vi "Proiecr_MDA.vi"() -> ()   [LabVIEW 2019]
uses:
  <vilib>/Analysis/Matrix/Datatypes/RealMatrix.ctl
  <vilib>/robotics/Kinematics/DH Kinematic Parameters.ctl
  <vilib>/robotics/Kinematics/Link/Joint Type.ctl
  <vilib>/robotics/Kinematics/NI_Kinematics.lvlib
  <vilib>/robotics/Kinematics/Link/NI_Robotics_Link.lvclass
  <vilib>/Analysis/Matrix/NI_Matrix.lvlib
panel:
  out "3D Picture":refnum<vi>(3d-picture)
  in  "j6":dbl(slide) scale=0.0..6.2831
  in  "j5":dbl(slide) scale=-1.5707..1.5707
  in  "j4":dbl(slide) scale=0.0..6.2831
  in  "j3":dbl(slide) scale=-2.5..2.5
  in  "j2":dbl(slide) scale=-2.17..2.17
  in  "j1":dbl(slide) scale=0.0..6.2831
  out "array to string":string
  in  "index":dbl
  out "Array":cluster{string, "number of columns":i32}[](array[cluster])
  in  "stop":bool
  out "Translation Matrix":T1
  out "Rotation Matrix Fake":T1
  out "Orientation XYZ Fake":dbl[](array[numeric])
  in  "Debug":bool
  in  "?":enum32{"Configuration", "Manipulate", "Points"}(tab)
  in  "j6 L":dbl
  in  "j4 L":dbl
  in  "j5 L":dbl=-1.5707
  in  "j1 L":dbl
  in  "j2 L":dbl=-2.17
  in  "j3 L":dbl=-2.5
  in  "j6 U":dbl=6.2831
  in  "j4 U":dbl=6.2831
  in  "j5 U":dbl=1.5707
  in  "j1 U":dbl=6.2831
  in  "j2 U":dbl=2.17
  in  "j3 U":dbl=2.5
  in  "l1":dbl=1.3
  in  "l2":dbl=2.5
  in  "l3":dbl=1.25
  in  "l4":dbl=1.25
  in  "l5":dbl=1.0
  in  "base":dbl=0.9
  in  "Generate file":bool
  in  "Pause time (sec)":i64=1
  in  "End Spline":bool
  out "Select Trajectory":bool
  out "Loop activ":bool
  in  "Loop":bool
  out "Gripper Closed":bool
  in  "Activate Gripper":bool
  out "Active":bool
  out "End Point":bool
  out "Intermidiate Point":bool
  in  "Spline":bool
  in  "Circle":bool
  in  "Line":bool
  in  "Add Point":bool
  out "RX":dbl
  out "RY":dbl
  out "RZ":dbl
  out "X":dbl
  out "Y":dbl
  out "Z":dbl
  in  "Pause":bool
  out "Real Matrix":T1
  # "Dimensions of the manipulator"
  # "Arm"
  # "Wrist"
  # "Base"
  # "Limits of the joints"
  # "Joint 1"
  # "Joint 2"
  # "Joint 3"
  # "Upper\nLimit"
  # "Lower\nLimit"
  # "Joint 4"
  # "Joint 5"
  # "Joint 6"
  # "Upper\nLimit"
  # "Lower\nLimit"
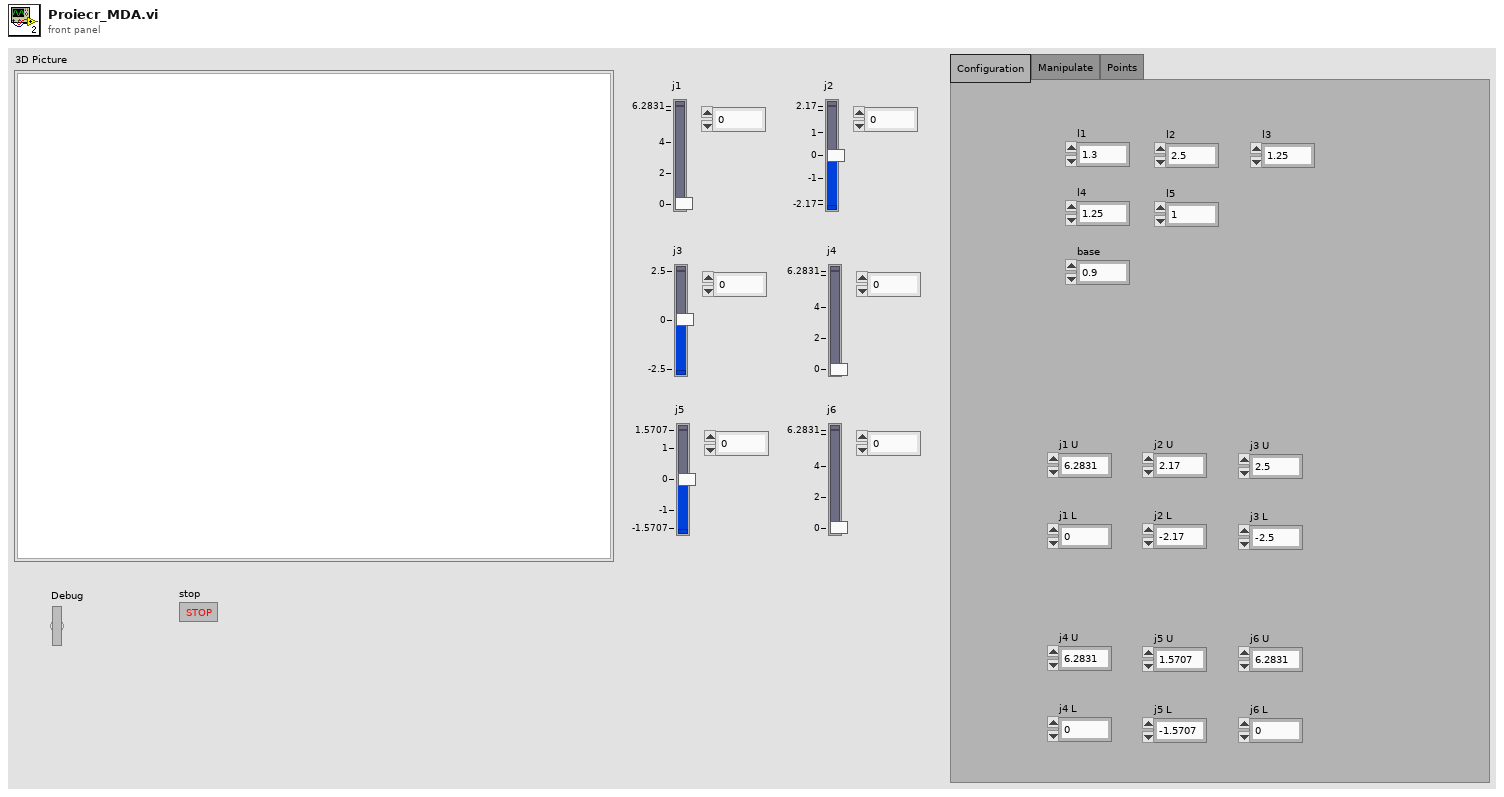
[diagram p1: front panel]
types:
  T1 = typedef "NI_Matrix.lvlib/RealMatrix.ctl" = dbl[][]
  T2 = enum16{"open", "replace", "create", "open or create", "replace or create", "replace or create with confirmation"}
  T3 = enum8{"Enabled", "Disabled", "Disabled and Grayed Out"}
  T4 = typedef "DH Kinematic Parameters.ctl" = cluster{"twist angle":dbl, "length":dbl, "rotation angle":dbl, "offset distance":dbl, "joint type":T5, "joint coordinate offset":dbl}
  T5 = typedef "NI_Robotics_Link.lvclass/Joint Type.ctl" = enum16{"Revolute", "Prismatic"}
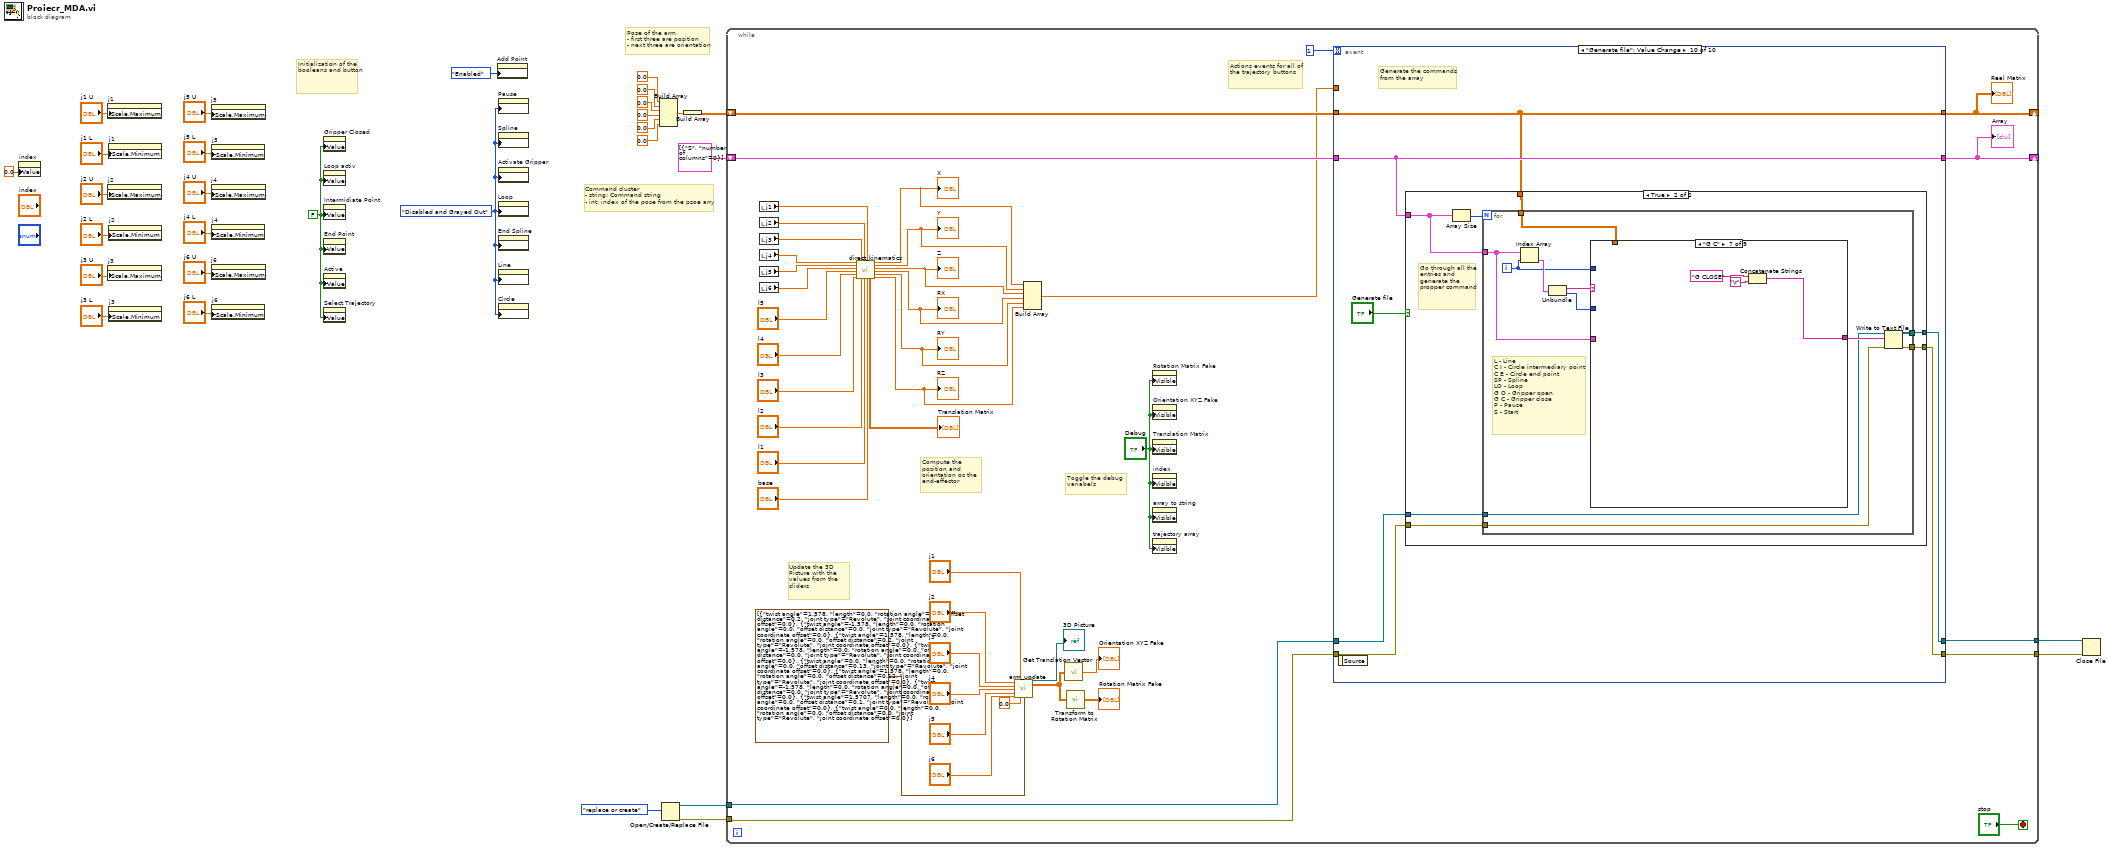
[diagram p0: block diagram]
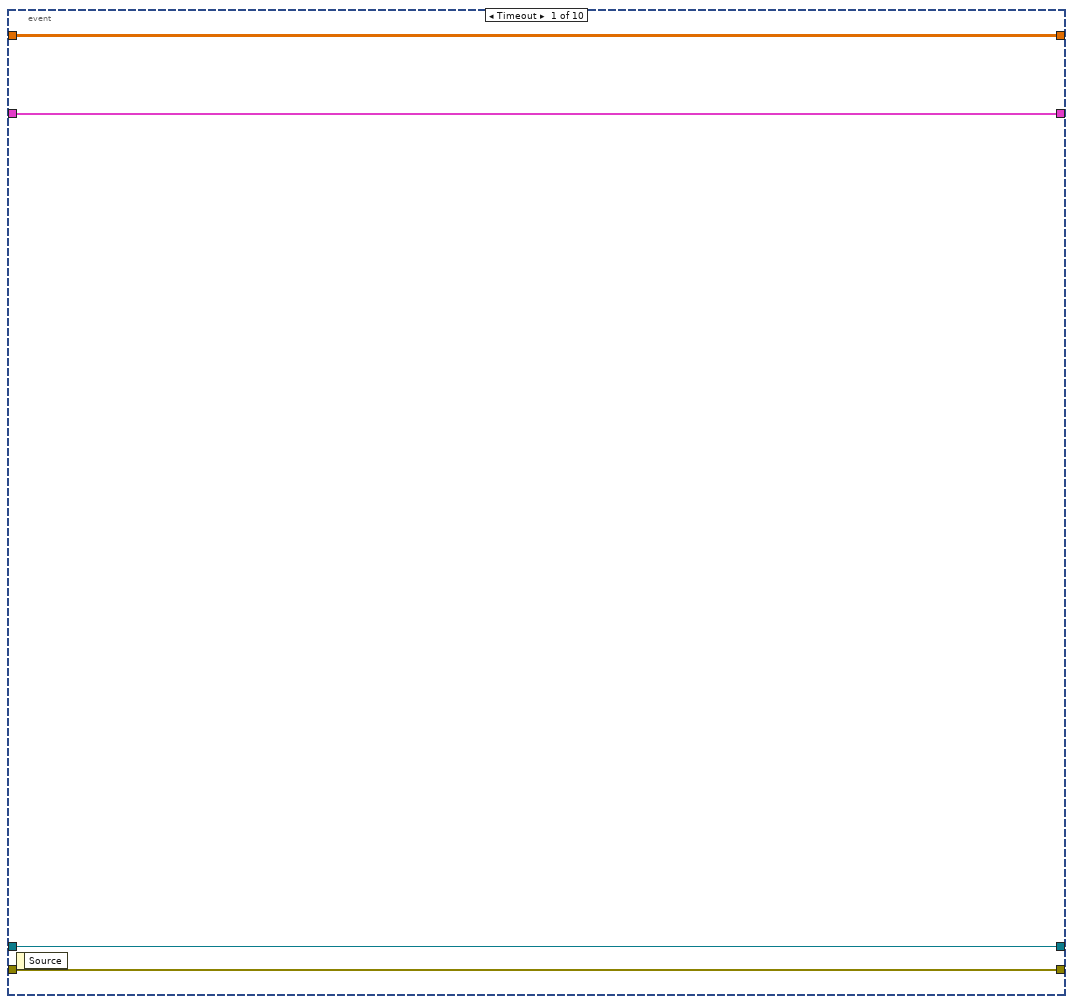
[diagram p2: hidden frame]
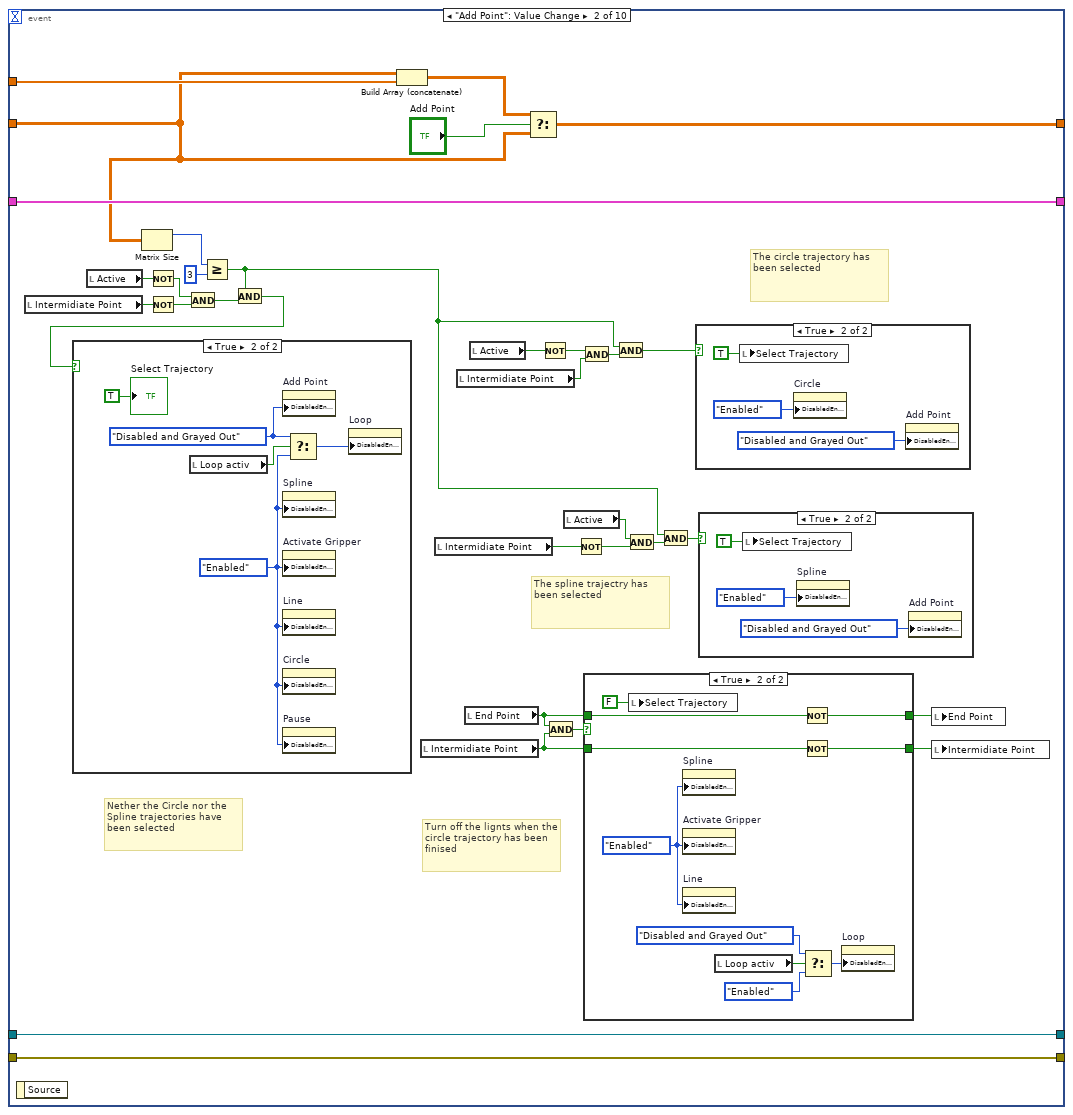
[diagram p3: hidden frame]
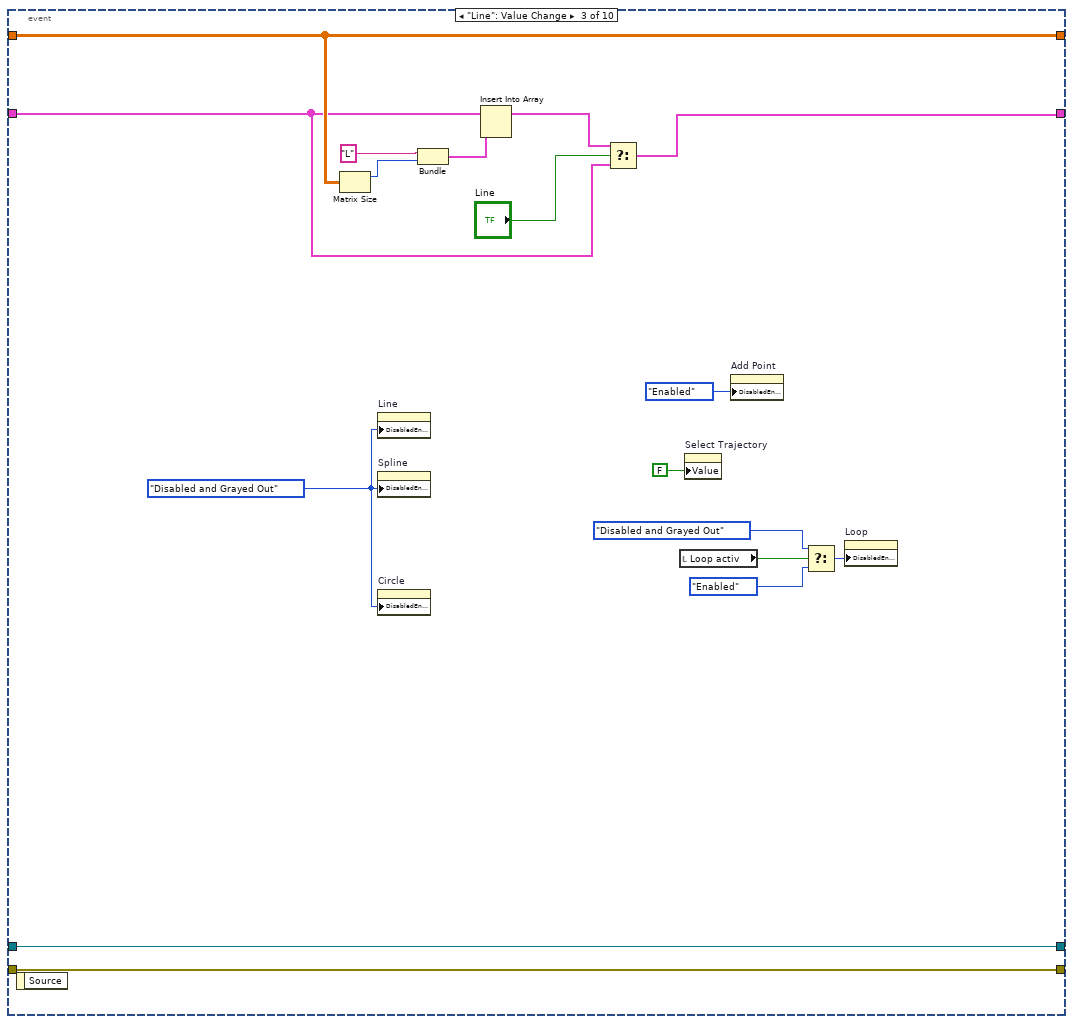
[diagram p8: hidden frame]
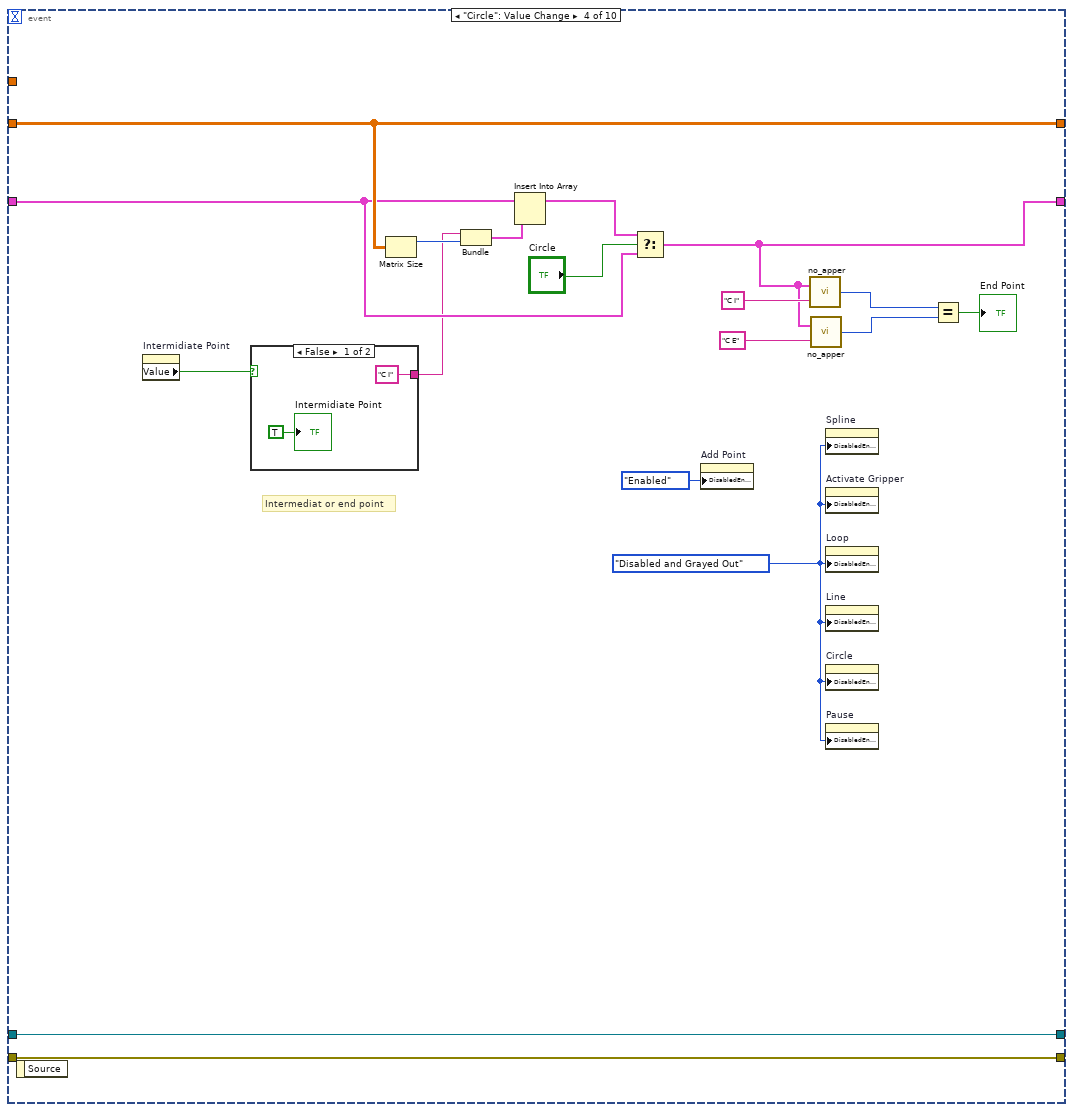
[diagram p9: hidden frame]
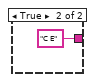
[diagram p10: hidden frame]
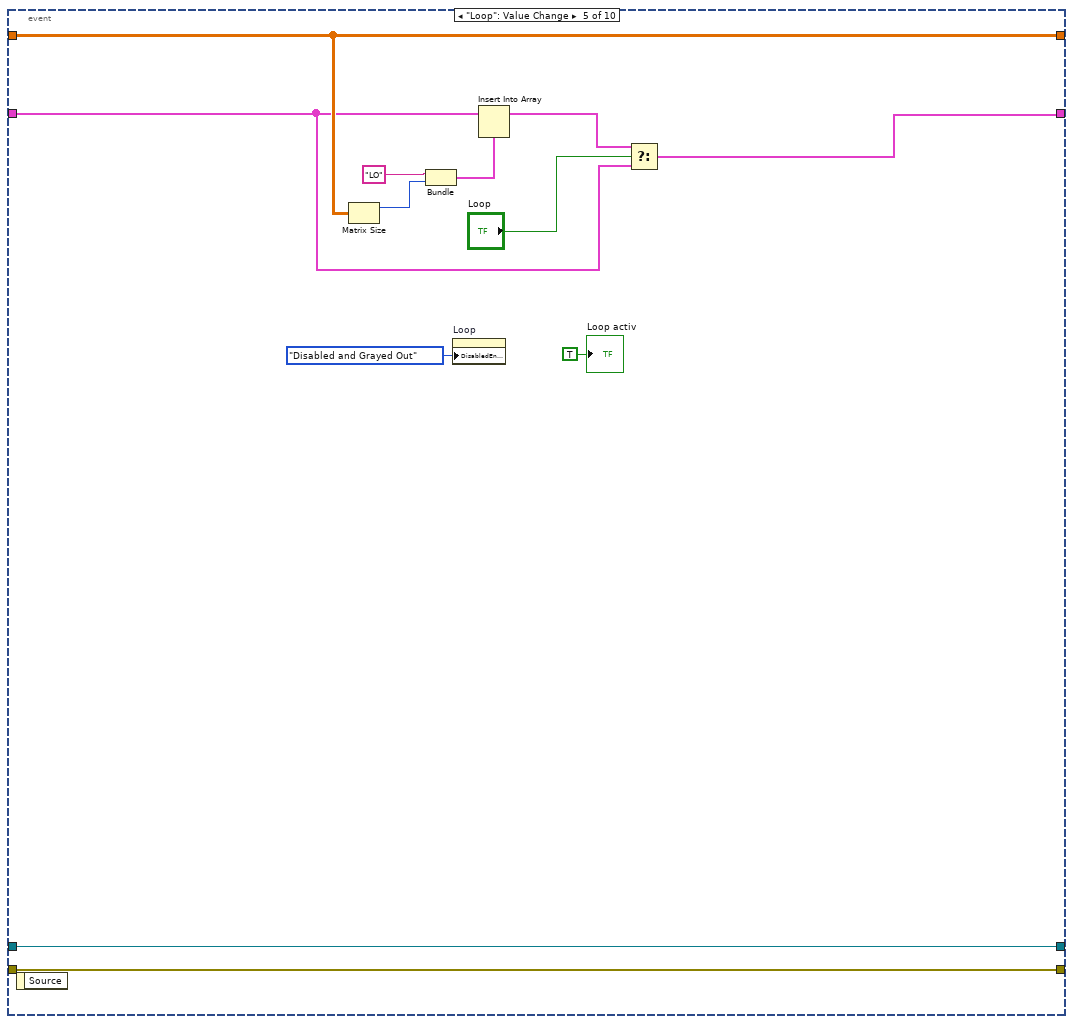
[diagram p11: hidden frame]
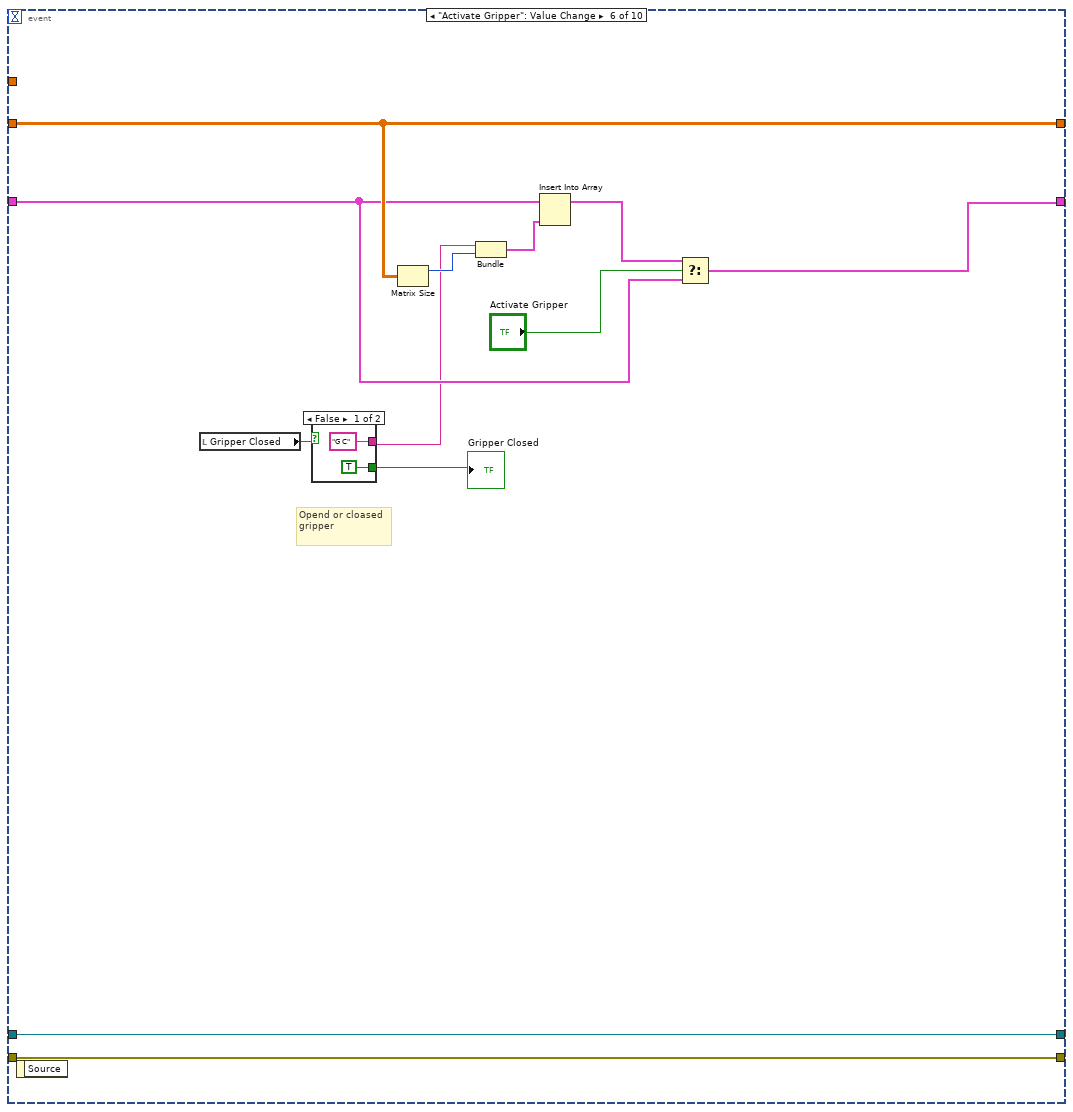
[diagram p12: hidden frame]
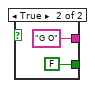
[diagram p13: hidden frame]
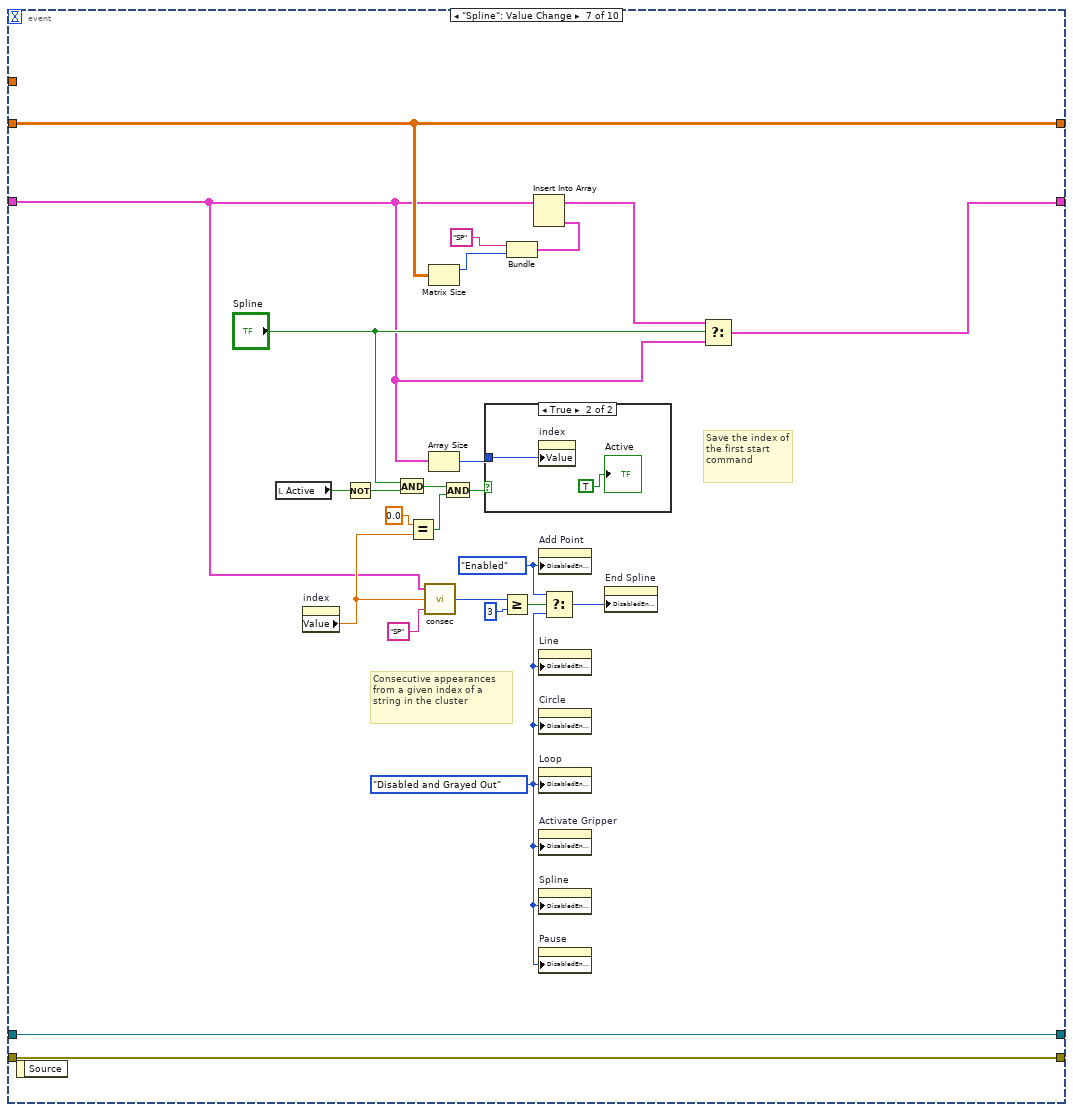
[diagram p14: hidden frame]
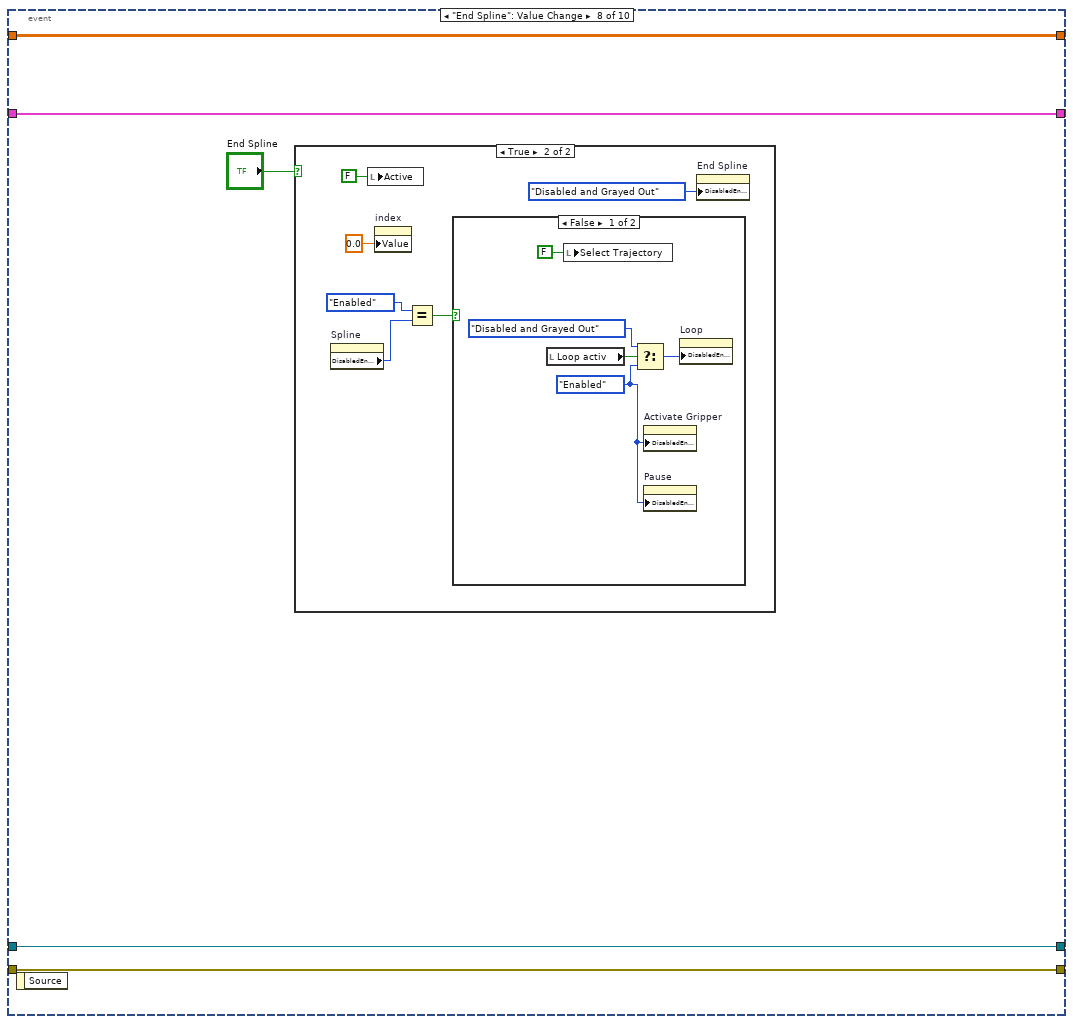
[diagram p16: hidden frame]
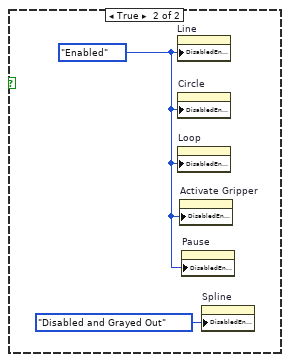
[diagram p18: hidden frame]
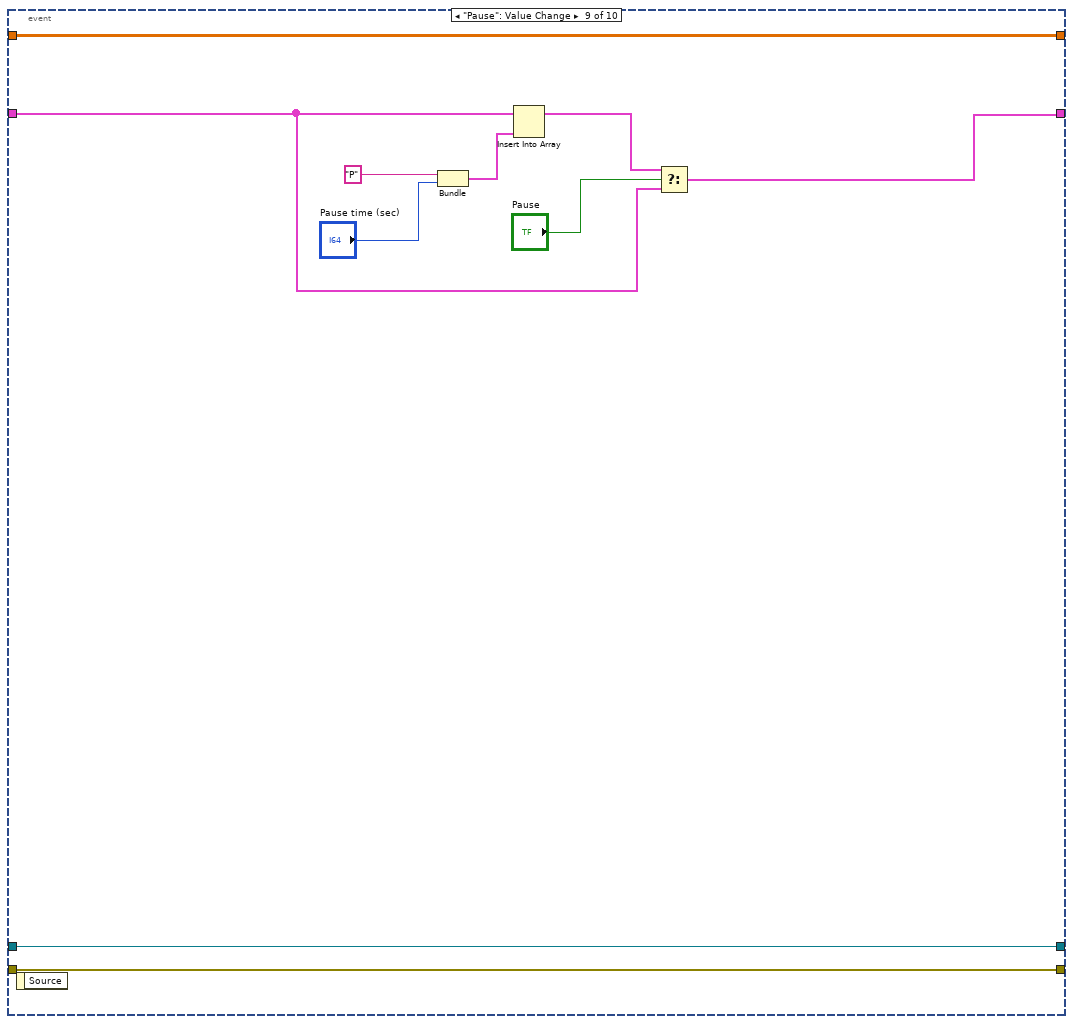
[diagram p19: hidden frame]
diagram:
  w2 = FALSE
  w8 = T3."Disabled and Grayed Out" ("Disabled")
  # "Command cluster \n- string: Command string \n- int: index of the pose from the psoe arry"
  # "Pose of the arm\n- first three are position \n- next three are orientation"
  # "Initialization of the booleans and button"
  n1 = property on="index" class="DigNum (strict)"("Value"=0.0 ("index")) -> ()  [unwired: 2 in, 2 out]
  n2 = property on="j1" class="Slide (strict)"("Scale.Maximum"="j1 U") -> ()  [unwired: 2 in, 2 out]
  n3 = property on="j2" class="Slide (strict)"("Scale.Maximum"="j2 U") -> ()  [unwired: 2 in, 2 out]
  n4 = property on="j3" class="Slide (strict)"("Scale.Maximum"="j3 U") -> ()  [unwired: 2 in, 2 out]
  n5 = property on="j1" class="Slide (strict)"("Scale.Minimum"="j1 L") -> ()  [unwired: 2 in, 2 out]
  n6 = property on="j2" class="Slide (strict)"("Scale.Minimum"="j2 L") -> ()  [unwired: 2 in, 2 out]
  n7 = property on="j3" class="Slide (strict)"("Scale.Minimum"="j3 L") -> ()  [unwired: 2 in, 2 out]
  n8 = property on="j5" class="Slide (strict)"("Scale.Maximum"="j5 U") -> ()  [unwired: 2 in, 2 out]
  n9 = property on="j4" class="Slide (strict)"("Scale.Maximum"="j4 U") -> ()  [unwired: 2 in, 2 out]
  n10 = property on="j6" class="Slide (strict)"("Scale.Maximum"="j6 U") -> ()  [unwired: 2 in, 2 out]
  n11 = property on="j5" class="Slide (strict)"("Scale.Minimum"="j5 L") -> ()  [unwired: 2 in, 2 out]
  n12 = property on="j4" class="Slide (strict)"("Scale.Minimum"="j4 L") -> ()  [unwired: 2 in, 2 out]
  n13 = property on="j6" class="Slide (strict)"("Scale.Minimum"="j6 L") -> ()  [unwired: 2 in, 2 out]
  n14 = property on="Gripper Closed" class="Bool (strict)"("Value"=w2) -> ()  [unwired: 2 in, 2 out]
  n15 = property on="Loop activ" class="Bool (strict)"("Value"=w2) -> ()  [unwired: 2 in, 2 out]
  n16 = property on="Intermidiate Point" class="Bool (strict)"("Value"=w2) -> ()  [unwired: 2 in, 2 out]
  n17 = property on="End Point" class="Bool (strict)"("Value"=w2) -> ()  [unwired: 2 in, 2 out]
  n18 = property on="Active" class="Bool (strict)"("Value"=w2) -> ()  [unwired: 2 in, 2 out]
  n19 = property on="Select Trajectory" class="Bool (strict)"("Value"=w2) -> ()  [unwired: 2 in, 2 out]
  n20 = property on="Add Point" class="Bool (strict)"("DisabledEnum"=T3."Enabled" ("Disabled")) -> ()  [unwired: 2 in, 2 out]
  n21 = property on="Pause" class="Bool (strict)"("DisabledEnum"=w8) -> ()  [unwired: 2 in, 2 out]
  n22 = property on="Spline" class="Bool (strict)"("DisabledEnum"=w8) -> ()  [unwired: 2 in, 2 out]
  n23 = property on="Activate Gripper" class="Bool"("DisabledEnum"=w8) -> ()  [unwired: 2 in, 2 out]
  n24 = property on="Loop" class="Bool (strict)"("DisabledEnum"=w8) -> ()  [unwired: 2 in, 2 out]
  n25 = property on="End Spline" class="Bool (strict)"("DisabledEnum"=w8) -> ()  [unwired: 2 in, 2 out]
  n26 = property on="Line" class="Bool (strict)"("DisabledEnum"=w8) -> ()  [unwired: 2 in, 2 out]
  n27 = property on="Circle" class="Bool (strict)"("DisabledEnum"=w8) -> ()  [unwired: 2 in, 2 out]
  n28 = Build Array(0.0 ("element"), 0.0 ("element"), 0.0 ("element"), 0.0 ("element"), 0.0 ("element"), 0.0 ("element")) -> (w13:dbl[])
  n29 = Open/Create/Replace File(operation (0:open)=T2."replace or create") -> (refnum out=w4:refnum<file>, error out=w5:errorcluster)  [unwired: 5 in, 1 out]
  n30 = Build Array(w13) -> (w12:T1)
  n31 = while {
    shift-right: [w62] -> _
    shift-left: w12 -> [w69]
    shift-right: [w67] -> _
    shift-left: cluster{string, "number of columns":i32}[] [{"S", "number of columns"=0}] -> [w68]
    tunnel: [w66] -> w7
    tunnel: [w65] -> w6
    tunnel: w5 -> [w64]
    tunnel: w4 -> [w63]
    stop <- "stop" stop-if-true
    # "Actions events for all of the trajectory buttons"
    # "Toggle the debug variabels"
    # "Update the 3D Picture with the values from the sliders"
    # "Compute the position and orientation oc the end-effector"
    n32 = local read "j1"() -> (w52:dbl)
    n33 = local read "j2"() -> (w51:dbl)
    n34 = local read "j3"() -> (w50:dbl)
    n35 = local read "j4"() -> (w49:dbl)
    n36 = local read "j5"() -> (w48:dbl)
    n37 = local read "j6"() -> (w47:dbl)
    n38 = call "direct_kinematics.vi"("j4"=w49, "j5"=w48, "j6"=w47, "l5"="l5", "l4"="l4", "l3"="l3", "j3"=w50, "l2"="l2", "j2"=w51, "l1"="l1", "j1"=w52, "base"="base") -> ("Translation Matrix"=→"Translation Matrix":T1, "X"=w39:dbl, "Y"=w38:dbl, "Z"=w37:dbl, "RX"=w36:dbl, "RY"=w35:dbl, "RZ"=w34:dbl)  [unwired: 1 in]
    "RX" <- w36
    "RY" <- w35
    "RZ" <- w34
    "X" <- w39
    "Y" <- w38
    "Z" <- w37
    n39 = call "arm_update.vi"("j2"="j2", "j1"="j1", "j3"="j3", "j4"="j4", "j5"="j5", "j6"="j6", "element"=0.0, "kinematic parameters"=T4[] [{"twist angle"=1.578, "length"=0.0, "rotation angle"=0.0, "offset distance"=0.2, "joint type"=enum."Revolute", "joint coordinate offset"=0.0}, {"twist angle"=-1.578, "length"=0.0, "rotation angle"=0.0, "offset distance"=0.0, "joint type"=enum."Revolute", "joint coordinate offset"=0.0}, {"twist angle"=1.578, "length"=0.0, "rotation angle"=0.0, "offset distance"=0.2, "joint type"=enum."Revolute", "joint coordinate offset"=0.0}, {"twist angle"=-1.578, "length"=0.0, "rotation angle"=0.0, "offset distance"=0.0, "joint type"=enum."Revolute", "joint coordinate offset"=0.0}, {"twist angle"=0.0, "length"=0.0, "rotation angle"=0.0, "offset distance"=0.13, "joint type"=enum."Revolute", "joint coordinate offset"=0.0}, {"twist angle"=1.578, "length"=0.0, "rotation angle"=0.0, "offset distance"=0.12, "joint type"=enum."Revolute", "joint coordinate offset"=0.0}, {"twist angle"=-1.578, "length"=0.0, "rotation angle"=0.0, "offset distance"=0.0, "joint type"=enum."Revolute", "joint coordinate offset"=0.0}, {"twist angle"=1.5707, "length"=0.0, "rotation angle"=0.0, "offset distance"=0.1, "joint type"=enum."Revolute", "joint coordinate offset"=0.0}, {"twist angle"=0.0, "length"=0.0, "rotation angle"=0.0, "offset distance"=0.0, "joint type"=enum."Revolute", "joint coordinate offset"=0.0}]) -> ("SceneObject out"=→"3D Picture":refnum<vi>, "end effector transform"=w53:T1)  [unwired: 6 in]
    n40 = Build Array(w39, w38, w37, w36, w35, w34) -> (w33:dbl[])
    n41 = call <vilib>:"Get Translation Vector.vi"("transform"=w53) -> ("translation vector"=→"Orientation XYZ Fake":dbl[])
    n42 = call <vilib>:"Transform to Rotation Matrix.vi"("transform"=w53) -> ("rotation matrix"=→"Rotation Matrix Fake":T1)
    n43 = property on="Rotation Matrix Fake" class="Arr (strict)"("Visible"="Debug") -> ()  [unwired: 2 in, 2 out]
    n44 = property on="Orientation XYZ Fake" class="Arr (strict)"("Visible"="Debug") -> ()  [unwired: 2 in, 2 out]
    n45 = property on="Translation Matrix" class="Arr (strict)"("Visible"="Debug") -> ()  [unwired: 2 in, 2 out]
    n46 = property on="index" class="DigNum (strict)"("Visible"="Debug") -> ()  [unwired: 2 in, 2 out]
    n47 = property on="array to string" class="Str"("Visible"="Debug") -> ()  [unwired: 2 in, 2 out]
    n48 = property on="trajectory array" class="Arr (strict)"("Visible"="Debug") -> ()  [unwired: 2 in, 2 out]
    n49 = event shown="[9] \"Generate file\": Value Change" {
      selector: _ -> [_ _ _ _ _ _ _ _ _ _]
      dyn-events: _ -> [_ _ _ _ _ _ _ _ _ _]
      timeout: 1 -> [_ _ _ _ _ _ _ _ _ _]
      tunnel: w33 -> [_ w109 _ _ _ _ _ _ _ _]
      tunnel: [w77 w106 w148 w164 w177 w190 w220 w230 w249 w259] -> w62
      tunnel: w69 -> [w77 w78 w148 w164 w177 w190 w220 w230 w249 w259]
      tunnel: w68 -> [w76 w103 w141 w162 w176 w189 w200 w229 w251 w260]
      tunnel: [w76 w103 w142 w150 w174 w191 w221 w229 w250 w260] -> w67
      tunnel: [w74 w79 w133 w157 w171 w183 w201 w226 w244 w258] -> w66
      tunnel: [w75 w80 w134 w158 w172 w184 w202 w227 w245 w257] -> w65
      tunnel: w64 -> [w74 w79 w133 w157 w171 w183 w201 w226 w244 w256]
      tunnel: w63 -> [w75 w80 w134 w158 w172 w184 w202 w227 w245 w255]
      event Timeout {
        n50 = event-data() -> ()  [unwired: 1 in, 1 out]
      }
      event "Add Point": Value Change {
        # "Turn off the lignts when the circle trajectory has been finised"
        # "The spline trajectry has been selected"
        # "The circle trajectory has been selected"
        # "Nether the Circle nor the Spline trajectories have been selected"
        n51 = event-data() -> ()  [unwired: 1 in, 1 out]
        n52 = local read "Intermidiate Point"() -> (w97:bool)
        n53 = local read "Active"() -> (w95:bool)
        n54 = Matrix Size(0:w78) -> (1:w105:i32)  [unwired: 1 out]
        n55 = Not(x=w95) -> (.not. x?=w94:bool)
        n56 = Not(x=w97) -> (.not. x?=w96:bool)
        n57 = And(x=w94, y=w96) -> (x .and. y?=w98:bool)
        n58 = Greater Or Equal?(x=w105, y=3) -> (x >= y?=w83:bool)
        n59 = And(x=w83, y=w98) -> (x .and. y?=w99:bool)
        n60 = case shown="True" w99 {
          frame False {
          }
          frame True {
            w118 = T3."Disabled and Grayed Out" ("Disabled")
            w116 = T3."Enabled" ("Disabled")
            n61 = local read "Loop activ"() -> (w119:bool)
            n62 = property on="Add Point" class="Bool (strict)"("DisabledEnum"=w118) -> ()  [unwired: 2 in, 2 out]
            n63 = property on="Spline" class="Bool (strict)"("DisabledEnum"=w116) -> ()  [unwired: 2 in, 2 out]
            n64 = property on="Activate Gripper" class="Bool"("DisabledEnum"=w116) -> ()  [unwired: 2 in, 2 out]
            n65 = property on="Line" class="Bool (strict)"("DisabledEnum"=w116) -> ()  [unwired: 2 in, 2 out]
            n66 = property on="Circle" class="Bool (strict)"("DisabledEnum"=w116) -> ()  [unwired: 2 in, 2 out]
            n67 = property on="Pause" class="Bool (strict)"("DisabledEnum"=w116) -> ()  [unwired: 2 in, 2 out]
            n68 = Select(t=w118, s=w119, f=w116) -> (s? t:f=w117:T3)
            n69 = property on="Loop" class="Bool (strict)"("DisabledEnum"=w117) -> ()  [unwired: 2 in, 2 out]
            "Select Trajectory" <- TRUE ("Select Trajectory")
          }
        }
        n70 = Build Array (concatenate)(w78, w109) -> (w107:T1)
        n71 = local read "Intermidiate Point"() -> (w82:bool)
        n72 = local read "Intermidiate Point"() -> (w88:bool)
        n73 = local read "Intermidiate Point"() -> (w91:bool)
        n74 = local read "End Point"() -> (w81:bool)
        n75 = local read "Active"() -> (w93:bool)
        n76 = Select(t=w107, s="Add Point", f=w78) -> (s? t:f=w106:T1)
        n77 = Not(x=w93) -> (.not. x?=w92:bool)
        n78 = And(x=w81, y=w82) -> (x .and. y?=w102:bool)
        n79 = local read "Active"() -> (w87:bool)
        n80 = Not(x=w88) -> (.not. x?=w86:bool)
        n81 = And(x=w92, y=w91) -> (x .and. y?=w90:bool)
        n82 = case shown="True" w102 {
          tunnel: w82 -> [w122 w132]
          tunnel: w81 -> [w121 w131]
          tunnel: [w121 w130] -> w101
          tunnel: [w122 w129] -> w100
          frame False {
          }
          frame True {
            w127 = T3."Enabled" ("Disabled")
            n83 = local write "Select Trajectory"(FALSE) -> ()
            n84 = property on="Spline" class="Bool (strict)"("DisabledEnum"=w127) -> ()  [unwired: 2 in, 2 out]
            n85 = property on="Activate Gripper" class="Bool"("DisabledEnum"=w127) -> ()  [unwired: 2 in, 2 out]
            n86 = property on="Line" class="Bool (strict)"("DisabledEnum"=w127) -> ()  [unwired: 2 in, 2 out]
            n87 = local read "Loop activ"() -> (w126:bool)
            n88 = Not(x=w131) -> (.not. x?=w130:bool)
            n89 = Not(x=w132) -> (.not. x?=w129:bool)
            n90 = Select(t=T3."Disabled and Grayed Out" ("Disabled"), s=w126, f=T3."Enabled" ("Disabled")) -> (s? t:f=w123:T3)
            n91 = property on="Loop" class="Bool (strict)"("DisabledEnum"=w123) -> ()  [unwired: 2 in, 2 out]
          }
        }
        n92 = And(x=w83, y=w90) -> (x .and. y?=w89:bool)
        n93 = And(x=w87, y=w86) -> (x .and. y?=w84:bool)
        n94 = And(x=w83, y=w84) -> (x .and. y?=w85:bool)
        n95 = case shown="True" w89 {
          frame False {
          }
          frame True {
            n96 = local write "Select Trajectory"(TRUE ("Select Trajectory")) -> ()
            n97 = property on="Circle" class="Bool (strict)"("DisabledEnum"=T3."Enabled" ("Disabled")) -> ()  [unwired: 2 in, 2 out]
            n98 = property on="Add Point" class="Bool (strict)"("DisabledEnum"=T3."Disabled and Grayed Out" ("Disabled")) -> ()  [unwired: 2 in, 2 out]
          }
        }
        n99 = case shown="True" w85 {
          frame False {
          }
          frame True {
            n100 = local write "Select Trajectory"(TRUE ("Select Trajectory")) -> ()
            n101 = property on="Spline" class="Bool (strict)"("DisabledEnum"=T3."Enabled" ("Disabled")) -> ()  [unwired: 2 in, 2 out]
            n102 = property on="Add Point" class="Bool (strict)"("DisabledEnum"=T3."Disabled and Grayed Out" ("Disabled")) -> ()  [unwired: 2 in, 2 out]
          }
        }
        n103 = local write "End Point"(w101) -> ()
        n104 = local write "Intermidiate Point"(w100) -> ()
      }
      event "Line": Value Change {
        w135 = T3."Disabled and Grayed Out" ("Disabled")
        n105 = event-data() -> ()  [unwired: 1 in, 1 out]
        n106 = Matrix Size(0:w148) -> (1:w147:i32)  [unwired: 1 out]
        n107 = property on="Line" class="Bool (strict)"("DisabledEnum"=w135) -> ()  [unwired: 2 in, 2 out]
        n108 = property on="Spline" class="Bool (strict)"("DisabledEnum"=w135) -> ()  [unwired: 2 in, 2 out]
        n109 = property on="Circle" class="Bool (strict)"("DisabledEnum"=w135) -> ()  [unwired: 2 in, 2 out]
        n110 = Bundle("L", "number of columns"=w147) -> (w145:cluster{string, "number of columns":i32})  [unwired: 1 in]
        n111 = Insert Into Array(array=w141, new element=w145) -> (w143:cluster{string, "number of columns":i32}[])  [unwired: 1 in]
        n112 = Select(t=w143, s="Line", f=w141) -> (s? t:f=w142:cluster{string, "number of columns":i32}[])
        n113 = local read "Loop activ"() -> (w139:bool)
        n114 = property on="Select Trajectory" class="Bool (strict)"("Value"=FALSE ("Select Trajectory")) -> ()  [unwired: 2 in, 2 out]
        n115 = property on="Add Point" class="Bool (strict)"("DisabledEnum"=T3."Enabled" ("Disabled")) -> ()  [unwired: 2 in, 2 out]
        n116 = Select(t=T3."Disabled and Grayed Out" ("Disabled"), s=w139, f=T3."Enabled" ("Disabled")) -> (s? t:f=w137:T3)
        n117 = property on="Loop" class="Bool (strict)"("DisabledEnum"=w137) -> ()  [unwired: 2 in, 2 out]
      }
      event "Circle": Value Change {
        w159 = T3."Disabled and Grayed Out" ("Disabled")
        # "Intermediat or end point"
        n118 = event-data() -> ()  [unwired: 1 in, 1 out]
        n119 = property on="Intermidiate Point" class="Bool (strict)"() -> ("Value"=w156:bool)  [unwired: 2 in, 2 out]
        n120 = case shown="False" w156 {
          tunnel: ["C I" "C E"] -> w155
          frame False {
            "Intermidiate Point" <- TRUE ("Intermidiate Point")
          }
          frame True {
          }
        }
        n121 = Matrix Size(0:w164) -> (1:w167:i32)  [unwired: 1 out]
        n122 = Bundle(w155, "number of columns"=w167) -> (w166:cluster{string, "number of columns":i32})  [unwired: 1 in]
        n123 = Insert Into Array(array=w162, new element=w166) -> (w165:cluster{string, "number of columns":i32}[])  [unwired: 1 in]
        n124 = Select(t=w165, s="Circle", f=w162) -> (s? t:f=w150:cluster{string, "number of columns":i32}[])
        n125 = property on="Add Point" class="Bool (strict)"("DisabledEnum"=T3."Enabled" ("Disabled")) -> ()  [unwired: 2 in, 2 out]
        n126 = call "no_apper.vi"("String"="C I", "Array"=w150) -> ("Numeric"=w152:i32)
        n127 = call "no_apper.vi"("String"="C E", "Array"=w150) -> ("Numeric"=w151:i32)
        n128 = property on="Spline" class="Bool (strict)"("DisabledEnum"=w159) -> ()  [unwired: 2 in, 2 out]
        n129 = property on="Activate Gripper" class="Bool"("DisabledEnum"=w159) -> ()  [unwired: 2 in, 2 out]
        n130 = property on="Loop" class="Bool (strict)"("DisabledEnum"=w159) -> ()  [unwired: 2 in, 2 out]
        n131 = property on="Line" class="Bool (strict)"("DisabledEnum"=w159) -> ()  [unwired: 2 in, 2 out]
        n132 = property on="Circle" class="Bool (strict)"("DisabledEnum"=w159) -> ()  [unwired: 2 in, 2 out]
        n133 = property on="Pause" class="Bool (strict)"("DisabledEnum"=w159) -> ()  [unwired: 2 in, 2 out]
        n134 = Equal?(x=w152, y=w151) -> (x = y?=→"End Point":bool)
      }
      event "Loop": Value Change {
        n135 = event-data() -> ()  [unwired: 1 in, 1 out]
        n136 = Matrix Size(0:w177) -> (1:w180:i32)  [unwired: 1 out]
        n137 = Bundle("LO", "number of columns"=w180) -> (w179:cluster{string, "number of columns":i32})  [unwired: 1 in]
        n138 = property on="Loop" class="Bool (strict)"("DisabledEnum"=T3."Disabled and Grayed Out" ("Disabled")) -> ()  [unwired: 2 in, 2 out]
        n139 = Insert Into Array(array=w176, new element=w179) -> (w178:cluster{string, "number of columns":i32}[])  [unwired: 1 in]
        n140 = Select(t=w178, s="Loop", f=w176) -> (s? t:f=w174:cluster{string, "number of columns":i32}[])
        "Loop activ" <- TRUE ("Loop activ")
      }
      event "Activate Gripper": Value Change {
        # "Opend or cloased gripper"
        n141 = event-data() -> ()  [unwired: 1 in, 1 out]
        n142 = local read "Gripper Closed"() -> (w185:bool)
        n143 = case shown="False" w185 {
          tunnel: [TRUE FALSE] -> w188
          tunnel: ["G C" "G O"] -> w187
          frame False {
          }
          frame True {
          }
        }
        "Gripper Closed" <- w188
        n144 = Matrix Size(0:w190) -> (1:w194:i32)  [unwired: 1 out]
        n145 = Bundle(w187, "number of columns"=w194) -> (w193:cluster{string, "number of columns":i32})  [unwired: 1 in]
        n146 = Insert Into Array(array=w189, new element=w193) -> (w192:cluster{string, "number of columns":i32}[])  [unwired: 1 in]
        n147 = Select(t=w192, s="Activate Gripper", f=w189) -> (s? t:f=w191:cluster{string, "number of columns":i32}[])
      }
      event "Spline": Value Change {
        w203 = T3."Disabled and Grayed Out" ("Disabled")
        w205 = T3."Enabled" ("Disabled")
        # "Save the index of the first start command"
        # "Consecutive appearances from a given index of a string in the cluster"
        n148 = event-data() -> ()  [unwired: 1 in, 1 out]
        n149 = local read "Active"() -> (w212:bool)
        n150 = property on="index" class="DigNum (strict)"() -> ("Value"=w208:dbl)  [unwired: 2 in, 2 out]
        n151 = Not(x=w212) -> (.not. x?=w211:bool)
        n152 = And(x="Spline", y=w211) -> (x .and. y?=w215:bool)
        n153 = Equal?(x=0.0, y=w208) -> (x = y?=w214:bool)
        n154 = call "consec.vi"("String"="SP", "Start"=w208, "Array"=w200) -> ("Numeric"=w210:i32)
        n155 = Matrix Size(0:w220) -> (1:w217:i32)  [unwired: 1 out]
        n156 = Array Size(array=w200) -> (size(s)=w204:i32)
        n157 = And(x=w215, y=w214) -> (x .and. y?=w216:bool)
        n158 = case shown="True" w216 {
          tunnel: w204 -> [_ w225]
          frame False {
          }
          frame True {
            n159 = property on="index" class="DigNum (strict)"("Value"=w225) -> ()  [unwired: 2 in, 2 out]
            "Active" <- TRUE ("Active")
          }
        }
        n160 = Greater Or Equal?(x=w210, y=3) -> (x >= y?=w207:bool)
        n161 = Bundle("SP", "number of columns"=w217) -> (w223:cluster{string, "number of columns":i32})  [unwired: 1 in]
        n162 = Insert Into Array(array=w200, new element=w223) -> (w222:cluster{string, "number of columns":i32}[])  [unwired: 1 in]
        n163 = property on="Add Point" class="Bool (strict)"("DisabledEnum"=w205) -> ()  [unwired: 2 in, 2 out]
        n164 = property on="Line" class="Bool (strict)"("DisabledEnum"=w203) -> ()  [unwired: 2 in, 2 out]
        n165 = property on="Circle" class="Bool (strict)"("DisabledEnum"=w203) -> ()  [unwired: 2 in, 2 out]
        n166 = property on="Loop" class="Bool (strict)"("DisabledEnum"=w203) -> ()  [unwired: 2 in, 2 out]
        n167 = property on="Activate Gripper" class="Bool"("DisabledEnum"=w203) -> ()  [unwired: 2 in, 2 out]
        n168 = property on="Spline" class="Bool (strict)"("DisabledEnum"=w203) -> ()  [unwired: 2 in, 2 out]
        n169 = property on="Pause" class="Bool (strict)"("DisabledEnum"=w203) -> ()  [unwired: 2 in, 2 out]
        n170 = Select(t=w205, s=w207, f=w203) -> (s? t:f=w206:T3)
        n171 = property on="End Spline" class="Bool (strict)"("DisabledEnum"=w206) -> ()  [unwired: 2 in, 2 out]
        n172 = Select(t=w222, s="Spline", f=w200) -> (s? t:f=w221:cluster{string, "number of columns":i32}[])
      }
      event "End Spline": Value Change {
        n173 = event-data() -> ()  [unwired: 1 in, 1 out]
        n174 = case shown="True" "End Spline" {
          frame False {
          }
          frame True {
            n175 = property on="Spline" class="Bool (strict)"() -> ("DisabledEnum"=w232:T3)  [unwired: 2 in, 2 out]
            n176 = local write "Active"(FALSE ("Active")) -> ()
            n177 = property on="index" class="DigNum (strict)"("Value"=0.0 ("index")) -> ()  [unwired: 2 in, 2 out]
            n178 = Equal?(x=T3."Enabled" ("Disabled"), y=w232) -> (x = y?=w231:bool)
            n179 = case shown="False" w231 {
              frame False {
                w237 = T3."Enabled" ("Disabled")
                n180 = local read "Loop activ"() -> (w239:bool)
                n181 = local write "Select Trajectory"(FALSE ("Select Trajectory")) -> ()
                n182 = Select(t=T3."Disabled and Grayed Out" ("Disabled"), s=w239, f=w237) -> (s? t:f=w240:T3)
                n183 = property on="Activate Gripper" class="Bool"("DisabledEnum"=w237) -> ()  [unwired: 2 in, 2 out]
                n184 = property on="Pause" class="Bool (strict)"("DisabledEnum"=w237) -> ()  [unwired: 2 in, 2 out]
                n185 = property on="Loop" class="Bool (strict)"("DisabledEnum"=w240) -> ()  [unwired: 2 in, 2 out]
              }
              frame True {
                w243 = T3."Enabled" ("Disabled")
                n186 = property on="Line" class="Bool (strict)"("DisabledEnum"=w243) -> ()  [unwired: 2 in, 2 out]
                n187 = property on="Circle" class="Bool (strict)"("DisabledEnum"=w243) -> ()  [unwired: 2 in, 2 out]
                n188 = property on="Loop" class="Bool (strict)"("DisabledEnum"=w243) -> ()  [unwired: 2 in, 2 out]
                n189 = property on="Activate Gripper" class="Bool"("DisabledEnum"=w243) -> ()  [unwired: 2 in, 2 out]
                n190 = property on="Pause" class="Bool (strict)"("DisabledEnum"=w243) -> ()  [unwired: 2 in, 2 out]
                n191 = property on="Spline" class="Bool (strict)"("DisabledEnum"=T3."Disabled and Grayed Out" ("Disabled")) -> ()  [unwired: 2 in, 2 out]
              }
            }
            n192 = property on="End Spline" class="Bool (strict)"("DisabledEnum"=T3."Disabled and Grayed Out" ("Disabled")) -> ()  [unwired: 2 in, 2 out]
          }
        }
      }
      event "Pause": Value Change {
        n193 = event-data() -> ()  [unwired: 1 in, 1 out]
        n194 = Bundle("P", "Pause time (sec)"="Pause time (sec)") -> (w247:cluster{string, "Pause time (sec)":i64})  [unwired: 1 in]
        n195 = Insert Into Array(array=w251, new element=w247) -> (w252:cluster{string, "number of columns":i32}[])  [unwired: 1 in]
        n196 = Select(t=w252, s="Pause", f=w251) -> (s? t:f=w250:cluster{string, "number of columns":i32}[])
      }
      event "Generate file": Value Change {
        # "Generate the commands from the array"
        n197 = event-data() -> ()  [unwired: 1 in, 1 out]
        n198 = case shown="True" "Generate file" {
          tunnel: w260 -> [_ w263]
          tunnel: w259 -> [_ w269]
          tunnel: [w261 w268] -> w258
          tunnel: [w262 w267] -> w257
          tunnel: w256 -> [w261 w266]
          tunnel: w255 -> [w262 w265]
          frame False {
          }
          frame True {
            # "Go through all the entries and generate the propper command"
            n199 = Array Size(array=w263) -> (size(s)=w264:i32)
            n200 = for {
              N: w264 -> [_]
              tunnel: [w277] -> w267
              tunnel: [w276] -> w268
              tunnel: w263 -> [w270]
              tunnel: w269 -> [w275]
              tunnel: w266 -> [w274]
              tunnel: w265 -> [w273]
              i -> [w271]
              # "L - Line \nC I - Circle intermediary point\nC E - Circle end point\nSP - Spline\nLO - Loop\nG O - Gripper open \nG C - Gripper close\nP - Pause \nS - Start"
              n201 = Index Array(array=w270, index=w271) -> (element=w272:cluster{string, "number of columns":i32})
              n202 = Unbundle(w272) -> (w280:string, "number of columns"=w279:i32)
              n203 = case shown="\"G C\"" w280 {
                tunnel: w279 -> [w284 w290 w298 w307 _ _ _ w352 _]
                tunnel: [w285 w289 w297 w306 w339 w342 w345 w348 w354] -> w278
                tunnel: w275 -> [w287 w291 w299 w308 _ _ _ _ w355]
                tunnel: w271 -> [_ _ _ w312 _ _ _ _ _]
                tunnel: w270 -> [_ _ _ w305 _ _ _ _ _]
                frame "L" {
                  # "Convert an array to a singla string"
                  n204 = Decrement(x=w284) -> (x-1=w283:i32)
                  n205 = Index Array(array=w287, index (row)=w283) -> (element=w282:dbl[])  [unwired: 1 in]
                  n206 = call "array_to_string.vi"("Real Matrix"=w282) -> ("String"=w281:string)
                  "array to string" <- w281
                  n207 = Concatenate Strings("A LINE POSE ", w281, "\r") -> (w285:string)
                }
                frame "C I" {
                  n208 = Decrement(x=w290) -> (x-1=w294:i32)
                  n209 = Index Array(array=w291, index (row)=w294) -> (element=w295:dbl[])  [unwired: 1 in]
                  n210 = call "array_to_string.vi"("Real Matrix"=w295) -> ("String"=w296:string)
                  n211 = Concatenate Strings("A CIRCLE POSE_INTERMEDIARY ", w296, "\r") -> (w289:string)
                }
                frame "C E" {
                  n212 = Decrement(x=w298) -> (x-1=w302:i32)
                  n213 = Index Array(array=w299, index (row)=w302) -> (element=w303:dbl[])  [unwired: 1 in]
                  n214 = call "array_to_string.vi"("Real Matrix"=w303) -> ("String"=w304:string)
                  n215 = Concatenate Strings("A CIRCLE POSE_END ", w304, "\r") -> (w297:string)
                }
                frame "SP" {
                  n216 = Decrement(x=w312) -> (x-1=w313:i32)
                  n217 = Index Array(array=w305, index=w313) -> (element=w311:cluster{string, "number of columns":i32})
                  n218 = Unbundle(w311) -> (w310:string)  [unwired: 1 out]
                  n219 = Equal?(x=w310, y="SP") -> (x = y?=w309:bool)
                  n220 = case shown="False" w309 {
                    tunnel: w308 -> [w317 w333]
                    tunnel: w307 -> [w316 w332]
                    tunnel: [w324 w331] -> w306
                    tunnel: w305 -> [w328 _]
                    frame False {
                      # "Number of appearnces of a string in the cluster array"
                      n221 = Decrement(x=w316) -> (x-1=w321:i32)
                      n222 = Index Array(array=w317, index (row)=w321) -> (element=w322:dbl[])  [unwired: 1 in]
                      n223 = call "array_to_string.vi"("Real Matrix"=w322) -> ("String"=w318:string)
                      n224 = call "no_apper.vi"("String"="SP", "Array"=w328) -> ("Numeric"=w323:i32)
                      n225 = Concatenate Strings("A SPLINE POSE ", w318, "\r") -> (w315:string)
                      n226 = Number To Fractional String(number=w323, precision (6)=i16 0) -> (F-format string=w326:string)  [unwired: 2 in]
                      n227 = Concatenate Strings("A SPLINE COMMAND ", w326, "\r", w315) -> (w324:string)
                    }
                    frame True {
                      n228 = Decrement(x=w332) -> (x-1=w336:i32)
                      n229 = Index Array(array=w333, index (row)=w336) -> (element=w337:dbl[])  [unwired: 1 in]
                      n230 = call "array_to_string.vi"("Real Matrix"=w337) -> ("String"=w338:string)
                      n231 = Concatenate Strings("A SPLINE POSE ", w338, "\r") -> (w331:string)
                    }
                  }
                }
                frame "LO" {
                  n232 = Concatenate Strings("LOOP", "\r") -> (w339:string)
                }
                frame "G O" {
                  n233 = Concatenate Strings("G OPEN", "\r") -> (w342:string)
                }
                frame "G C" {
                  n234 = Concatenate Strings("G CLOSE", "\r") -> (w345:string)
                }
                frame "P" {
                  n235 = Number To Fractional String(number=w352, precision (6)=i16 0) -> (F-format string=w350:string)  [unwired: 2 in]
                  n236 = Concatenate Strings("A PAUSE SECONDS ", w350, "\r") -> (w348:string)
                }
                frame "S", Default {
                  n237 = Index Array(array=w355, index (row)=1) -> (element=w358:dbl[])  [unwired: 1 in]
                  n238 = call "array_to_string.vi"("Real Matrix"=w358) -> ("String"=w357:string)
                  n239 = Concatenate Strings("A PTP_COORD POSE ", w357, "\r") -> (w354:string)
                }
              }
              n240 = Write to Text File(file (use dialog)=w273, text=w278, error in=w274) -> (refnum out=w277:refnum<file>, error out=w276:errorcluster)  [unwired: 1 in, 1 out]
            }
          }
        }
      }
    }
    "Real Matrix" <- w62
    "Array" <- w67
  }
  n241 = Close File(refnum=w6, error in=w7) -> ()  [unwired: 2 out]
